vi "生成二维数组.vi"() -> ()   [LabVIEW 2014]
panel:
  out "维数 2":i32
  out "维数1":i32
  out "数组":dbl[][](array[numeric])
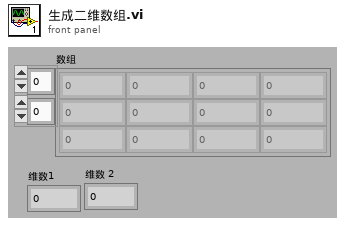
[diagram p1: front panel]
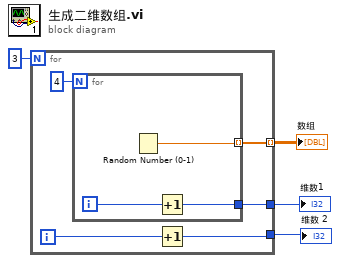
[diagram p0: block diagram]
diagram:
  n1 = for {
    N: 3 -> [_]
    tunnel: [w8] -> w3 mode=indexing
    tunnel: [w7] -> w2
    tunnel: [w5] -> w1
    i -> [w6]
    n2 = for {
      N: 4 -> [_]
      tunnel: [w12] -> w8 mode=indexing
      tunnel: [w10] -> w7
      i -> [w11]
      n3 = Random Number (0-1)() -> (number: 0 to 1=w12:dbl)
      n4 = Increment(x=w11) -> (x+1=w10:i32)
    }
    n5 = Increment(x=w6) -> (x+1=w5:i32)
  }
  "数组" <- w3
  "维数1" <- w2
  "维数 2" <- w1
